vi "Get Display String.vi"(11 "FP GT in":refnum<class "FP GT.lvclass">) -> (2 "Display String":string)   [LabVIEW 2018, in "FP GT.lvclass"]
uses:
  FP GT.lvclass
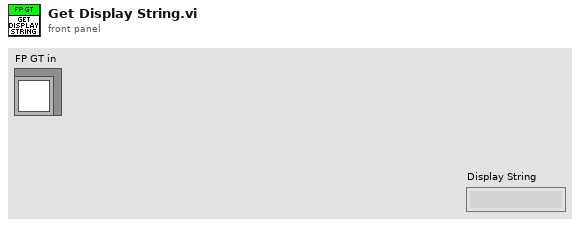
[diagram p1: front panel]
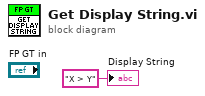
[diagram p0: block diagram]
diagram:
  "Display String" <- "X > Y" ("Display String")
